vi "LMS_FM_Demodulate_Example.vi"() -> ()   [LabVIEW 2018, in "LMS_LV_Drv.lvlib"]
uses:
  LMS_LV_Drv.lvlib
  Stream_ctl.ctl
  <vilib>/sound2/lvsound2.llb/Sampling Mode.ctl
  <vilib>/sound2/lvsound2.llb/Sound Data Format.ctl
  <vilib>/Analysis/3filter.llb/Filter Passband Type.ctl
  <vilib>/Analysis/1siggen.llb/Ramp Pattern by Samples.vi
  <vilib>/Analysis/2dsp.llb/Complex FFT.vi
  <vilib>/sound2/lvsound2.llb/Sound Output Write (DBL Single).vi
  <vilib>/Analysis/3filter.llb/Butterworth Filter (CDB).vi
  <vilib>/Analysis/2dsp.llb/Decimate (continuous, DBL).vi
  <vilib>/Analysis/NI_AALPro.lvlib
  <vilib>/Analysis/NI_AALBase.lvlib
panel:
  out "FM Spectrum":cluster{dbl[], dbl[]}[](graph)
  in  "Direction":u8(ring) items=["RX", "TX"]
  in  "Volume":dbl(knob)=0.8 min=0.0 max=2.0 step=0.1 scale=0.0..2.0
  in  "bandwidth":dbl=500000.0 format="%#_6p"
  out "EXIT":bool=TRUE
  in  "stop":bool
  in  "gain":u32=60
  in  "FM  Frequency":dbl=90500000.0 format="%#_6p"
  in  "chan":u64
  in  "stream":T1={"handle"=0, "isTx"=0, "channel"=0, "fifoSize"=100000, "throughputVsLatency"=1.0, "dataFmt"=0}
  out "LimeSDR_info":string="LimeSDR-USB, media=USB 3.0, module=FX3, serial=0009072C02891115, index=0"
  in  "Sample Rate":dbl=4000000.0 format="%#_6p"
  out "error out":errorcluster
  # "FM Demo"
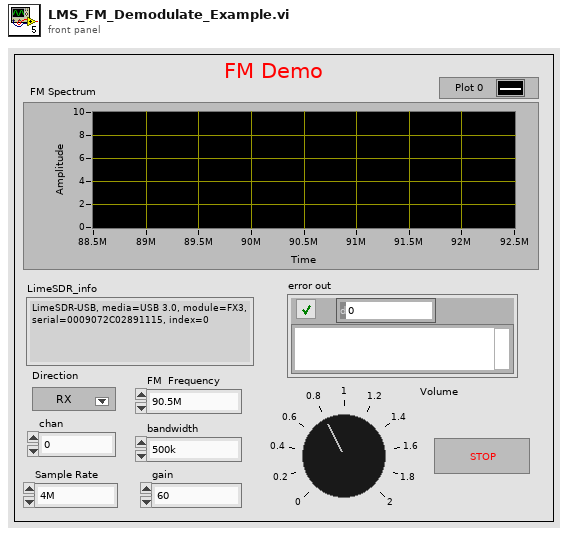
[diagram p1: front panel]
types:
  T1 = typedef "Stream_ctl.ctl" = cluster{"handle":u64, "isTx":u8, "channel":u32, "fifoSize":u32, "throughputVsLatency":dbl, "dataFmt":u32}
  T2 = typedef "Sound Data Format.ctl" = cluster{"sample rate (S/s)":dbl, "number of channels":i32, "bits per sample":i32}
  T3 = typedef "Sampling Mode.ctl" = i32
  T4 = typedef "Sound Output Task ID.ctl" = u32
  T5 = typedef "NI_AALBase.lvlib/Filter Passband Type.ctl" = enum32{"Lowpass", "Highpass", "Bandpass", "Bandstop"}
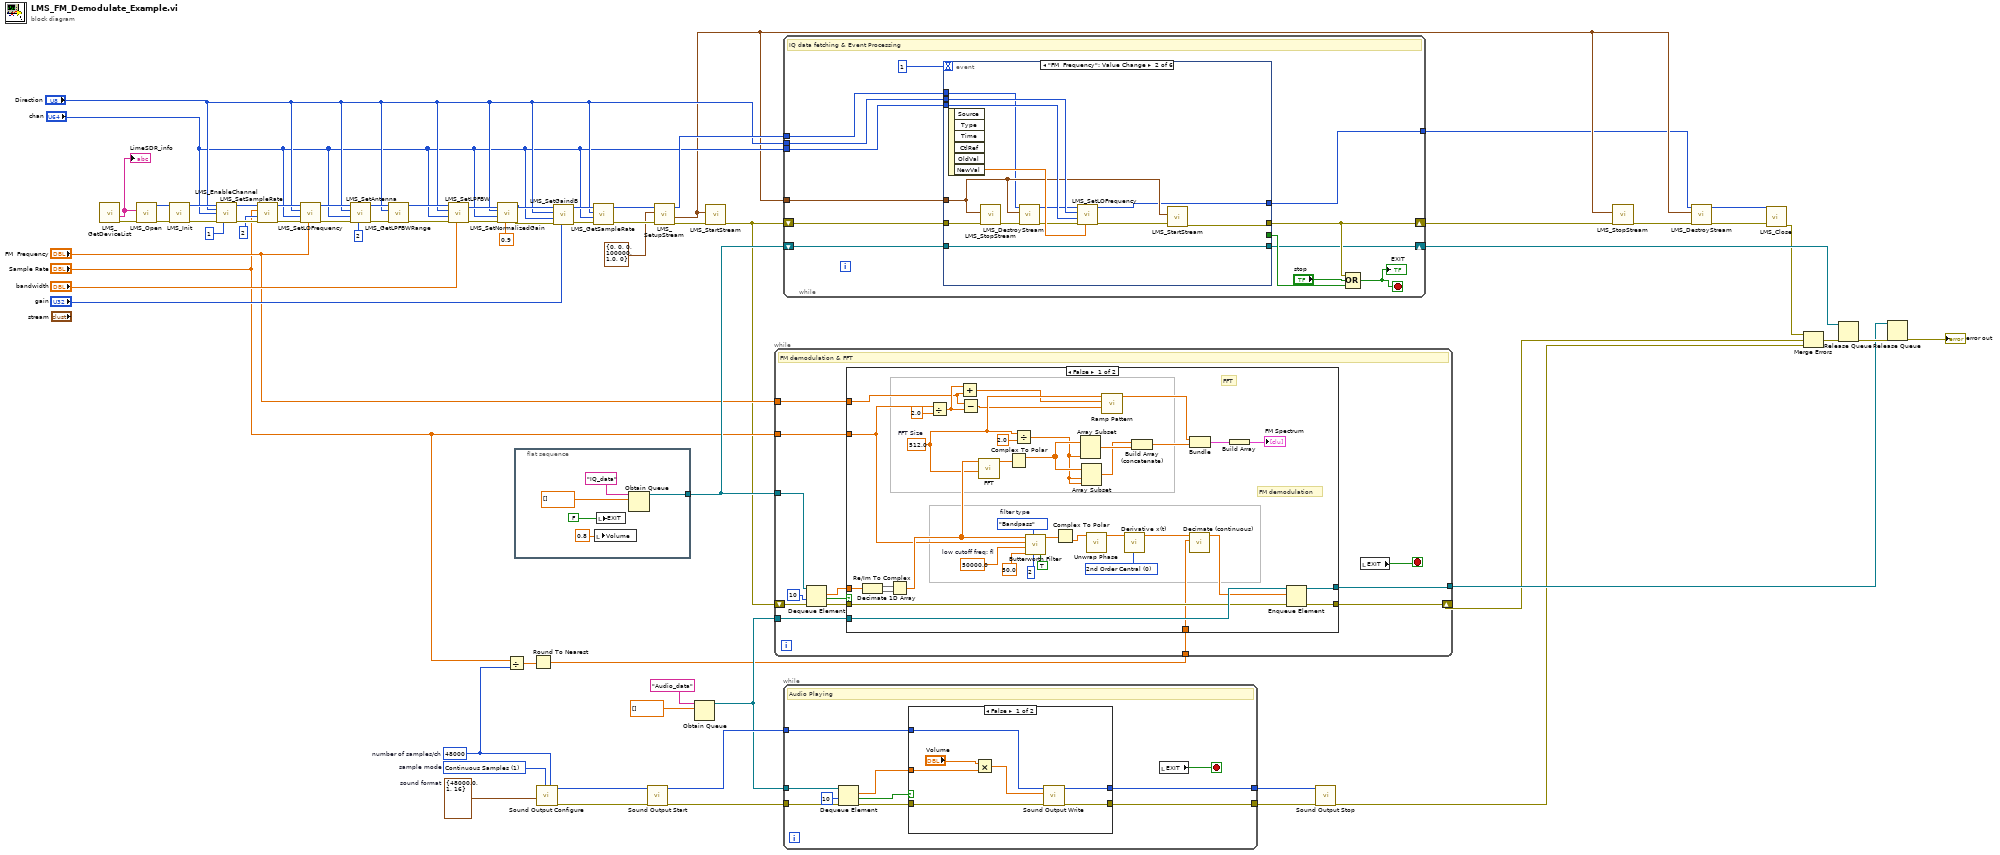
[diagram p0: block diagram]
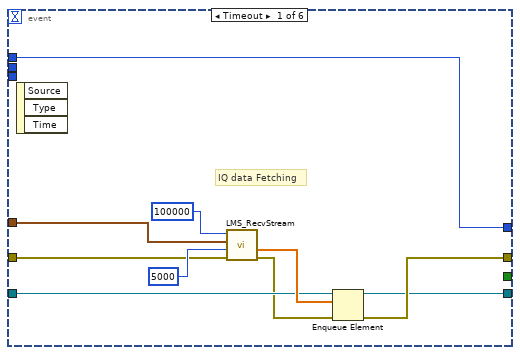
[diagram p4: hidden frame]
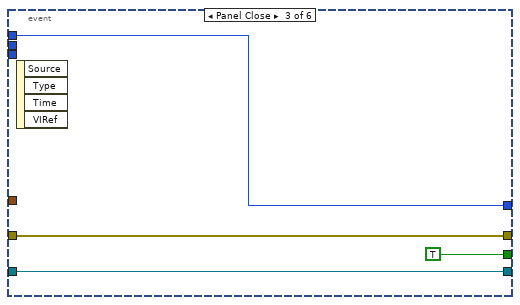
[diagram p5: hidden frame]
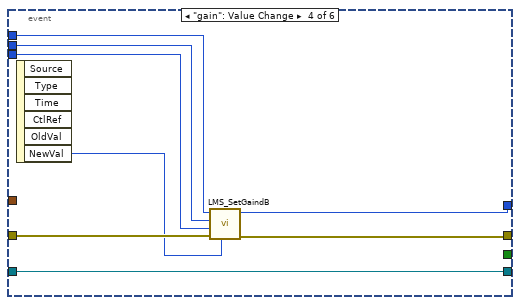
[diagram p6: hidden frame]
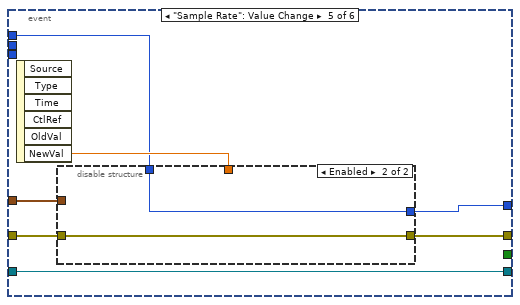
[diagram p7: hidden frame]
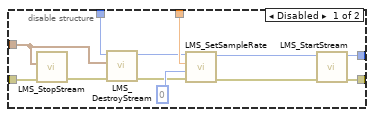
[diagram p8: hidden frame]
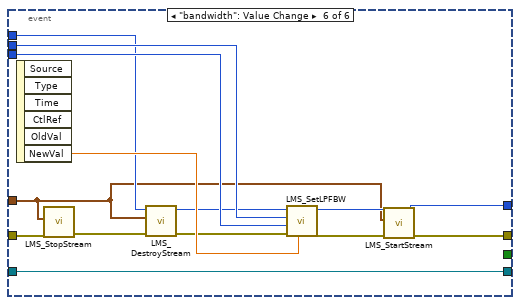
[diagram p9: hidden frame]
diagram:
  w9 = 48000  # number of samples/ch
  w30 = T2 {"sample rate (S/s)"=48000.0, "number of channels"=1, "bits per sample"=16}  # sound format
  w27 = T3 1 items=["Finite Samples", "Continuous Samples"]  # sample mode
  n1 = call "LMS_GetDeviceList.vi"() -> ("error out"=w67:errorcluster, "lms_info_str_t"=w66:string)  [unwired: 9 in, 1 out]
  "LimeSDR_info" <- w66
  n2 = call "LMS_Open.vi"("error in (no error)"=w67, "lms_info_str_t"=w66) -> ("error out"=w65:errorcluster, "device"=w64:i64)  [unwired: 8 in]
  n3 = call "LMS_Init.vi"("error in (no error)"=w65, "device_In"=w64) -> ("error out"=w54:errorcluster, "device_Out"=w55:i64)  [unwired: 8 in]
  n4 = call "LMS_EnableChannel.vi"("device_In"=w55, "dir_tx"="Direction", "chan"="chan", "error in (no error)"=w54, "enabled"=i8 1) -> ("device_Out"=w51:i64, "error out"=w52:errorcluster)  [unwired: 9 in]
  n5 = call "LMS_SetSampleRate.vi"("error in (no error)"=w52, "oversample"=u64 2, "rate"="Sample Rate", "device_In"=w51) -> ("error out"=w50:errorcluster, "device_Out"=w49:i64)  [unwired: 6 in]
  n6 = call "LMS_SetLOFrequency.vi"("frequency"="FM  Frequency", "error in (no error)"=w50, "chan"="chan", "dir_tx"="Direction", "device_In"=w49) -> ("error out"=w45:errorcluster, "device_Out"=w43:i64)  [unwired: 5 in]
  n7 = call "LMS_SetAntenna.vi"("index"=u64 2, "error in (no error)"=w45, "chan"="chan", "dir_tx"="Direction", "device_In"=w43) -> ("error out"=w44:errorcluster, "device_Out"=w42:i64)  [unwired: 5 in]
  n8 = call "LMS_GetLPFBWRange.vi"("error in (no error)"=w44, "dir_tx"="Direction", "device_In"=w42) -> ("error out"=w47:errorcluster, "device_Out"=w46:i64)  [unwired: 6 in, 1 out]
  n9 = call "LMS_SetLPFBW.vi"("bandwidth"="bandwidth", "error in (no error)"=w47, "chan"="chan", "dir_tx"="Direction", "device_In"=w46) -> ("error out"=w40:errorcluster, "device_Out"=w57:i64)  [unwired: 5 in]
  n10 = call "LMS_SetNormalizedGain.vi"("gain"=0.9, "error in (no error)"=w40, "chan"="chan", "dir_tx"="Direction", "device_In"=w57) -> ("error out"=w38:errorcluster, "device_Out"=w35:i64)  [unwired: 5 in]
  n11 = Divide(x="Sample Rate", y=w9) -> (x/y=w8:dbl)
  n12 = flat-sequence {
    tunnel: [w70] -> w36
    frame #0 {
      n13 = local write "Volume"(0.8 ("Volume")) -> ()
      n14 = local write "EXIT"(FALSE ("EXIT")) -> ()
      n15 = Obtain Queue(name (unnamed)="IQ_data", element data type=dbl[] [] ("samples")) -> (queue out=w70:refnum<queue>)  [unwired: 3 in, 2 out]
    }
  }
  n16 = Round To Nearest(number=w8) -> (nearest integer value=w7:dbl)
  n17 = call <vilib>:"Sound Output Configure.vi"("number of samples/ch"=w9, "sample mode"=w27, "sound format"=w30) -> ("error out"=w28:errorcluster, "task ID"=w29:T4)  [unwired: 7 in]
  n18 = call "LMS_SetGaindB.vi"("gain"="gain", "error in (no error)"=w38, "chan"="chan", "dir_tx"="Direction", "device_In"=w35) -> ("error out"=w17:errorcluster, "device_Out"=w16:i64)  [unwired: 5 in]
  n19 = call "LMS_GetSampleRate.vi"("error in (no error)"=w17, "chan"="chan", "dir_tx"="Direction", "device_In"=w16) -> ("error out"=w58:errorcluster, "device_Out"=w34:i64)  [unwired: 4 in, 2 out]
  n20 = call <vilib>:"Sound Output Start.vi"("error in (no error)"=w28, "task ID"=w29) -> ("error out"=w25:errorcluster, "task ID out"=w26:T4)  [unwired: 8 in]
  n21 = call "LMS_SetupStream.vi"("error in (no error)"=w58, "stream_In"=T1 {"handle"=0, "isTx"=0, "channel"=0, "fifoSize"=100000, "throughputVsLatency"=1.0, "dataFmt"=0} ("stream"), "device_In"=w34) -> ("error out"=w63:errorcluster, "steam_Out"=w2:T1, "device_Out"=w5:i64)  [unwired: 6 in]
  n22 = Obtain Queue(name (unnamed)="Audio_data", element data type=dbl[] [] ("Decimated Array")) -> (queue out=w13:refnum<queue>)  [unwired: 3 in, 2 out]
  n23 = call "LMS_StartStream.vi"("error in (no error)"=w63, "stream 2"=w2) -> ("error out"=w6:errorcluster)  [unwired: 9 in]
  n24 = while {
    tunnel: w36 -> [w85]
    tunnel: "Sample Rate" -> [w80]
    tunnel: w13 -> [w79]
    tunnel: [w78] -> w32
    shift-right: [w77] -> w21
    shift-left: w6 -> [w76]
    tunnel: "FM  Frequency" -> [w74]
    tunnel: w7 -> [w73]
    stop <- w82 stop-if-true
    # "FM demodulation & FFT"
    n25 = Dequeue Element(queue=w85, timeout in ms (-1)=10, error in (no error)=w76) -> (element=w83:dbl[], timed out?=w84:bool, error out=w75:errorcluster)  [unwired: 1 out]
    n26 = case shown="False" w84 {
      tunnel: w83 -> [w121 _]
      tunnel: w80 -> [w94 _]
      tunnel: w79 -> [w115 w124]
      tunnel: [w114 w124] -> w78
      tunnel: [w113 w123] -> w77
      tunnel: w75 -> [w109 w123]
      tunnel: w74 -> [w89 _]
      tunnel: w73 -> [w86 _]
      frame False {
        w91 = 512.0  # FFT Size
        w116 = u16 0 items=["2nd Order Central", "4th Order Central", "Forward", "Backward"] ("method")
        w117 = Filter_Passband_Type."Bandpass"  # filter type
        w111 = 50000.0  # low cutoff freq: fl
        # "FFT"
        # "FM demodulation"
        n27 = Decimate 1D Array(w121) -> (w120:dbl[], w119:dbl[])
        n28 = Re/Im To Complex(1:w119, 2:w120) -> (0:w104:cdb[])
        n29 = Divide(x=w94, y=2.0) -> (x/y=w90:dbl)
        n30 = Add(x=w90, y=w89) -> (x+y=w87:dbl)
        n31 = Subtract(x=w89, y=w90) -> (x-y=w88:dbl)
        n32 = call-poly <vilib>:"FFT.vi"("FFT size"=w91, "X"=w104) -> ("FFT {X}"=w122:cdb[])  [unwired: 8 in, 1 out]
        n33 = Complex To Polar(r * e^(i*theta)=w122) -> (r=w100:dbl[])  [unwired: 1 out]
        n34 = Divide(x=w91, y=2.0) -> (x/y=w98:dbl)
        n35 = call-poly <vilib>:"Butterworth Filter.vi"("init/cont (init:F)"=TRUE, "order"=2, "filter type"=w117, "low cutoff freq: fl"=50.0, "high cutoff freq: fh"=w111, "sampling freq: fs"=w94, "X"=w104) -> ("Filtered X"=w103:cdb[])  [unwired: 1 in, 1 out]
        n36 = Complex To Polar(r * e^(i*theta)=w103) -> (theta=w108:dbl[])  [unwired: 1 out]
        n37 = Array Subset(array=w100, length=w98) -> (w102:dbl[])  [unwired: 1 in]
        n38 = Array Subset(array=w100, index=w98, length=w98) -> (w101:dbl[])
        n39 = call <vilib>:"Unwrap Phase.vi"("Phase"=w108) -> ("Unwrapped Phase"=w112:dbl[])  [unwired: 9 in, 1 out]
        n40 = call-poly <vilib>:"Ramp Pattern.vi"("start"=w88, "end"=w87, "samples"=w91) -> ("Ramp Pattern"=w92:dbl[])  [unwired: 7 in, 1 out]
        n41 = call <vilib>:"Derivative x(t).vi"("method"=w116, "X"=w112) -> ("dX/dt"=w107:dbl[])  [unwired: 8 in, 1 out]
        n42 = Build Array (concatenate)(w101, w102) -> (w95:dbl[])
        n43 = call-poly <vilib>:"Decimate (continuous).vi"("decimating factor"=w86, "X"=w107) -> ("Decimated Array"=w105:dbl[])  [unwired: 8 in, 1 out]
        n44 = Bundle("Ramp Pattern"=w92, w95) -> (w97:cluster{"Ramp Pattern":dbl[], dbl[]})  [unwired: 1 in]
        n45 = Build Array(w97) -> (→"FM Spectrum":cluster{"Ramp Pattern":dbl[], dbl[]}[])
        n46 = Enqueue Element(queue=w115, element=w105, error in (no error)=w109) -> (queue out=w114:refnum<queue>, error out=w113:errorcluster)  [unwired: 1 in, 1 out]
      }
      frame True {
      }
    }
    n47 = local read "EXIT"() -> (w82:bool)
  }
  n48 = while {
    tunnel: w13 -> [w132]
    tunnel: w26 -> [w130]
    tunnel: w25 -> [w126]
    tunnel: [w128] -> w24
    tunnel: [w127] -> w23
    stop <- w134 stop-if-true
    # "Audio Playing"
    n49 = Dequeue Element(queue=w132, timeout in ms (-1)=10, error in (no error)=w126) -> (element=w129:dbl[], timed out?=w131:bool, error out=w125:errorcluster)  [unwired: 1 out]
    n50 = case shown="False" w131 {
      tunnel: w130 -> [w138 w143]
      tunnel: w129 -> [w136 _]
      tunnel: w125 -> [w141 w142]
      tunnel: [w140 w142] -> w128
      tunnel: [w139 w143] -> w127
      frame False {
        n51 = Multiply(x="Volume", y=w136) -> (x*y=w137:dbl[])
        n52 = call-poly <vilib>:"Sound Output Write.vi"("error in (no error)"=w141, "data"=w137, "task ID"=w138) -> ("error out"=w140:errorcluster, "task ID out"=w139:T4)  [unwired: 7 in]
      }
      frame True {
      }
    }
    n53 = local read "EXIT"() -> (w134:bool)
  }
  n54 = while {
    tunnel: w2 -> [w152]
    shift-right: [w150] -> w59
    shift-left: w6 -> [w147]
    shift-right: [w144] -> w56
    shift-left: w36 -> [w145]
    tunnel: w5 -> [w156]
    tunnel: "Direction" -> [w155]
    tunnel: "chan" -> [w154]
    tunnel: [w153] -> w1
    stop <- w151 stop-if-true
    # "IQ data fetching & Event Processing"
    n55 = event shown="[1] \"FM  Frequency\": Value Change" {
      selector: _ -> [_ _ _ _ _ _]
      dyn-events: _ -> [_ _ _ _ _ _]
      timeout: u32 1 ("milliseconds to wait") -> [_ _ _ _ _ _]
      tunnel: w147 -> [w163 w176 w183 w191 w195 w218]
      tunnel: w156 -> [w161 w169 w182 w189 w192 w217]
      tunnel: [w161 w168 w182 w188 w197 w223] -> w153
      tunnel: [w158 w175 w183 w190 w193 w213] -> w150
      tunnel: w155 -> [_ w179 _ w187 _ w222]
      tunnel: w154 -> [_ w178 _ w186 _ w221]
      tunnel: [_ _ TRUE _ _ _] -> w148
      tunnel: w152 -> [w162 w173 _ _ w194 w212]
      tunnel: w145 -> [w160 w174 w180 w184 w196 w220]
      tunnel: [w157 w174 w180 w184 w196 w220] -> w144
      event Timeout {
        # "IQ data Fetching"
        n56 = event-data() -> ()  [unwired: 1 in, 3 out]
        n57 = call "LMS_RecvStream.vi"("error in (no error)"=w163, "timeout_ms"=u32 5000, "stream"=w162, "sample_count"=u64 100000) -> ("error out"=w159:errorcluster, "samples"=w166:dbl[])  [unwired: 6 in]
        n58 = Enqueue Element(queue=w160, element=w166, error in (no error)=w159) -> (queue out=w157:refnum<queue>, error out=w158:errorcluster)  [unwired: 1 in, 1 out]
      }
      event "FM  Frequency": Value Change {
        n59 = event-data() -> ("NewVal"=w177:dbl)  [unwired: 1 in, 5 out]
        n60 = call "LMS_StopStream.vi"("error in (no error)"=w176, "stream"=w173) -> ("error out"=w172:errorcluster)  [unwired: 9 in]
        n61 = call "LMS_DestroyStream.vi"("error in (no error)"=w172, "stream"=w173, "device_In"=w169) -> ("error out"=w171:errorcluster, "device_Out"=w170:i64)  [unwired: 7 in]
        n62 = call "LMS_SetLOFrequency.vi"("frequency"=w177, "error in (no error)"=w171, "chan"=w178, "dir_tx"=w179, "device_In"=w170) -> ("error out"=w167:errorcluster, "device_Out"=w168:i64)  [unwired: 5 in]
        n63 = call "LMS_StartStream.vi"("error in (no error)"=w167, "stream 2"=w173) -> ("error out"=w175:errorcluster)  [unwired: 9 in]
      }
      event Panel Close {
        n64 = event-data() -> ()  [unwired: 1 in, 4 out]
      }
      event "gain": Value Change {
        n65 = event-data() -> ("NewVal"=w185:u32)  [unwired: 1 in, 5 out]
        n66 = call "LMS_SetGaindB.vi"("gain"=w185, "error in (no error)"=w191, "chan"=w186, "dir_tx"=w187, "device_In"=w189) -> ("error out"=w190:errorcluster, "device_Out"=w188:i64)  [unwired: 5 in]
      }
      event "Sample Rate": Value Change {
        n67 = event-data() -> ("NewVal"=w198:dbl)  [unwired: 1 in, 5 out]
        n68 = disable-structure shown="Enabled" {
          disable-tunnel: w198 -> [w208 _]
          disable-tunnel: [w207 w211] -> w197
          disable-tunnel: w195 -> [w206 w210]
          disable-tunnel: w194 -> [w204 _]
          disable-tunnel: [w201 w210] -> w193
          disable-tunnel: w192 -> [w200 w211]
          frame Disabled {
            n69 = call "LMS_StopStream.vi"("error in (no error)"=w206, "stream"=w204) -> ("error out"=w205:errorcluster)  [unwired: 9 in]
            n70 = call "LMS_DestroyStream.vi"("error in (no error)"=w205, "stream"=w204, "device_In"=w200) -> ("error out"=w203:errorcluster, "device_Out"=w199:i64)  [unwired: 7 in]
            n71 = call "LMS_SetSampleRate.vi"("error in (no error)"=w203, "oversample"=u64 0, "rate"=w208, "device_In"=w199) -> ("error out"=w202:errorcluster, "device_Out"=w207:i64)  [unwired: 6 in]
            n72 = call "LMS_StartStream.vi"("error in (no error)"=w202) -> ("error out"=w201:errorcluster)  [unwired: 10 in]
          }
          frame Enabled {
          }
        }
      }
      event "bandwidth": Value Change {
        n73 = event-data() -> ("NewVal"=w224:dbl)  [unwired: 1 in, 5 out]
        n74 = call "LMS_StopStream.vi"("error in (no error)"=w218, "stream"=w212) -> ("error out"=w219:errorcluster)  [unwired: 9 in]
        n75 = call "LMS_DestroyStream.vi"("error in (no error)"=w219, "stream"=w212, "device_In"=w217) -> ("error out"=w215:errorcluster, "device_Out"=w216:i64)  [unwired: 7 in]
        n76 = call "LMS_SetLPFBW.vi"("bandwidth"=w224, "error in (no error)"=w215, "chan"=w221, "dir_tx"=w222, "device_In"=w216) -> ("error out"=w214:errorcluster, "device_Out"=w223:i64)  [unwired: 5 in]
        n77 = call "LMS_StartStream.vi"("error in (no error)"=w214, "stream 2"=w212) -> ("error out"=w213:errorcluster)  [unwired: 9 in]
      }
    }
    n78 = Compound Arithmetic op=OR(w150, "stop", w148) -> (w151:bool)
    "EXIT" <- w151
  }
  n79 = call <vilib>:"Sound Output Stop.vi"("error in (no error)"=w24, "task ID"=w23) -> ("error out"=w20:errorcluster)  [unwired: 8 in, 1 out]
  n80 = call "LMS_StopStream.vi"("error in (no error)"=w59, "stream"=w2) -> ("error out"=w60:errorcluster)  [unwired: 9 in]
  n81 = call "LMS_DestroyStream.vi"("error in (no error)"=w60, "stream"=w2, "device_In"=w1) -> ("error out"=w62:errorcluster, "device_Out"=w61:i64)  [unwired: 7 in]
  n82 = call "LMS_Close.vi"("error in (no error)"=w62, "device_In"=w61) -> ("error out"=w22:errorcluster)  [unwired: 9 in]
  n83 = Merge Errors(w22, w21, w20) -> (w19:errorcluster)
  n84 = Release Queue(queue=w56, error in (no error)=w19) -> (error out=w33:errorcluster)  [unwired: 1 in, 2 out]
  n85 = Release Queue(queue=w32, error in (no error)=w33) -> (error out=→"error out":errorcluster)  [unwired: 1 in, 2 out]
